vi "Synchronize Manifold.vi"(8 "error in":errorcluster, 11 "Gantry in":refnum<class "Gantry.lvclass">) -> (0 "error out":errorcluster, 3 "Gantry out":refnum<class "Gantry.lvclass">)   [LabVIEW 2026, in "Gantry.lvclass"]
uses:
  Gantry.lvclass
  <vilib>/DAQmx/miscellaneous.llb/DAQmx Fill In Error Info.vi
  Gantry.lvclass/Gantry.ctl
  FlexWorktable/FlexWorktable.lvclass
  <vilib>/DAQmx/read.llb/DAQmx Read (Digital 1D Bool NChan 1Samp 1Line).vi
  GH2/GH2.lvclass
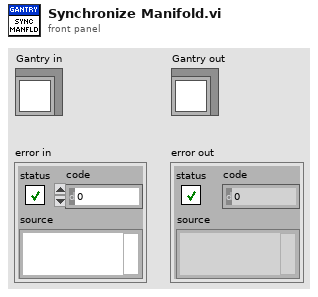
[diagram p1: front panel]
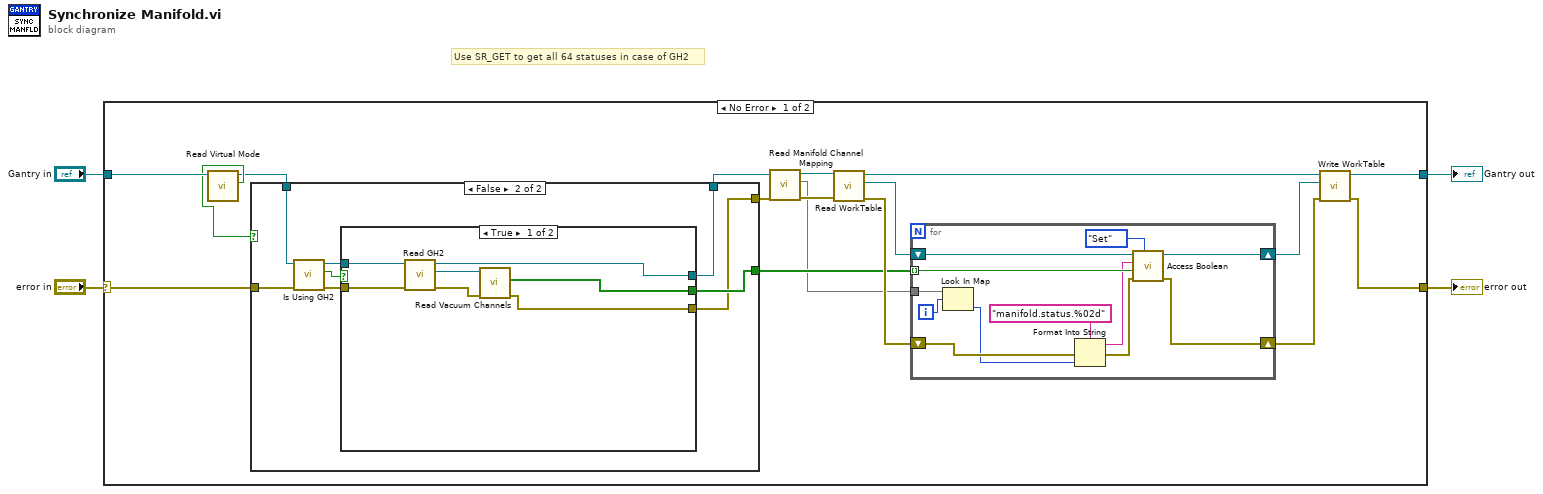
[diagram p0: block diagram]
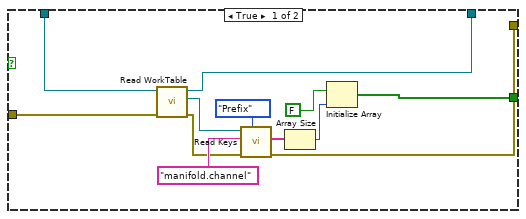
[diagram p2: hidden frame]
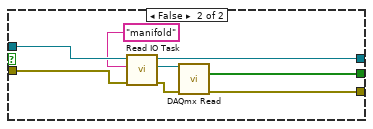
[diagram p3: hidden frame]
diagram:
  # "Use SR_GET to get all 64 statuses in case of GH2"
  n1 = case shown="No Error" "error in" {
    selector: "error in" -> [w5 w70]
    tunnel: [w20 w70] -> w3
    tunnel: [w21 w69] -> w1
    tunnel: "Gantry in" -> [w19 w69]
    frame No Error {
      n2 = call-dynamic "Read Virtual Mode.vi"("Gantry in"=w19) -> ("Is Virtual"=w13:bool, "Gantry out"=w6:refnum<class "Gantry.lvclass">)  [unwired: 7 in, 2 out]
      n3 = case shown="False" w13 {
        tunnel: [w32 w41] -> w10
        tunnel: [w23 w40] -> w8
        tunnel: w5 -> [w26 w36]
        tunnel: w6 -> [w27 w38]
        tunnel: [w25 w39] -> w7
        frame True {
          n4 = call-dynamic "Read WorkTable.vi"("error in"=w26, "Gantry Class in"=w27) -> ("error out"=w24:errorcluster, "Worktable"=w22:refnum<class "FlexWorktable.lvclass">, "Gantry Class out"=w25:refnum<class "Gantry.lvclass">)  [unwired: 7 in]
          n5 = call-dynamic "Read Keys.vi"("Prefix/Regex"=enum16{"Prefix", "Regex"}."Prefix", "error in (no error)"=w24, "Selector"="manifold.channel", "FlexWorktable in"=w22) -> ("error out"=w23:errorcluster, "Keys"=w29:string[])  [unwired: 5 in, 1 out]
          n6 = Array Size(array=w29) -> (size(s)=w28:i32)
          n7 = Initialize Array(FALSE, w28) -> (w32:bool[])
        }
        frame False {
          n8 = call "Is Using GH2.vi"("error in (no error)"=w36, "Gantry in"=w38) -> ("error out"=w35:errorcluster, "Using GH2"=w34:bool, "Gantry out"=w37:refnum<class "Gantry.lvclass">)  [unwired: 7 in]
          n9 = case shown="True" w34 {
            tunnel: [w43 w56] -> w41
            tunnel: [w44 w55] -> w40
            tunnel: w35 -> [w47 w54]
            tunnel: w37 -> [w48 w52]
            tunnel: [w42 w49] -> w39
            frame True {
              n10 = call "Read GH2.vi"("error in (no error)"=w47, "Gantry in"=w48) -> ("error out"=w45:errorcluster, "GH2.lvclass"=w46:refnum<class "GH2.lvclass">, "Gantry out"=w42:refnum<class "Gantry.lvclass">)  [unwired: 7 in]
              n11 = call "Read Vacuum Channels.vi"("error in (no error)"=w45, "GH2 in"=w46) -> ("error out"=w44:errorcluster, "Vacuum Channels"=w43:bool[])  [unwired: 7 in, 1 out]
            }
            frame False {
              n12 = call "Read IO Task.vi"("error in (no error)"=w54, "Task Name"="manifold", "Gantry in"=w52) -> ("error out"=w50:errorcluster, "task/channels in"=w53:refnum<k21>, "Gantry out"=w49:refnum<class "Gantry.lvclass">)  [unwired: 6 in]
              n13 = call-poly <vilib>:"DAQmx Read.vi"("task/channels in"=w53, "error in"=w50) -> ("data"=w56:bool[], "error out"=w55:errorcluster)  [unwired: 11 in, 1 out]
            }
          }
        }
      }
      n14 = call "Read Manifold Channel Mapping.vi"("error in (no error)"=w8, "Gantry in"=w7) -> ("error out"=w11:errorcluster, "Channel -> Port"=w9:map{i32, i32}, "Gantry out"=w12:refnum<class "Gantry.lvclass">)  [unwired: 6 in, 1 out]
      n15 = call-dynamic "Read WorkTable.vi"("error in"=w11, "Gantry Class in"=w12) -> ("error out"=w15:errorcluster, "Worktable"=w16:refnum<class "FlexWorktable.lvclass">, "Gantry Class out"=w14:refnum<class "Gantry.lvclass">)  [unwired: 7 in]
      n16 = for {
        tunnel: w10 -> [w65] mode=indexing
        shift-right: [w62] -> w17
        shift-left: w15 -> [w67]
        shift-right: [w61] -> w18
        shift-left: w16 -> [w66]
        tunnel: w9 -> [w59]
        i -> [w58]
        n17 = Look In Map(map=w59, key=w58) -> (value=w57:i32)  [unwired: 1 in, 1 out]
        n18 = Format Into String(format string="manifold.status.%02d", error in=w67, w57) -> (resulting string=w64:string, error out=w63:errorcluster)  [unwired: 1 in]
        n19 = call-dynamic "Access Boolean.vi"("Get/Set"=enum16{"Get", "Set"}."Set", "error in (no error)"=w63, "Value in"=w65, "Key"=w64, "FlexWorktable in"=w66) -> ("error out"=w62:errorcluster, "FlexWorktable out"=w61:refnum<class "FlexWorktable.lvclass">)  [unwired: 4 in, 1 out]
      }
      n20 = call-dynamic "Write WorkTable.vi"("error in (no error)"=w17, "FlexWorktable"=w18, "Gantry Class in"=w14) -> ("error out"=w20:errorcluster, "Gantry Class out"=w21:refnum<class "Gantry.lvclass">)  [unwired: 7 in]
    }
    frame Error {
    }
  }
  "error out" <- w3
  "Gantry out" <- w1
